vi "Meas 2 Target.vi"(7 "Cartesian Type":bool caption="CartesianType", 9 "LBCB 2  Data":T1, 10 "LBCB 1  Data":T1, 11 "Target":T2) -> (3 "Measured Value":T2)   [LabVIEW 2009]
uses:
  Target.ctl
  Data Access Objects/Metadata/LBCB Number.ctl
  Mixed Mode Cartesian Data.ctl
  Global Data/Cartesian Measurment Actions.ctl
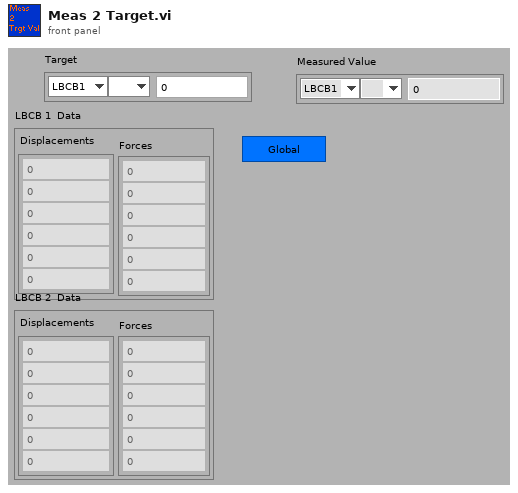
[diagram p1: front panel]
types:
  T1 = typedef "Mixed Mode Cartesian Data.ctl" = cluster{"Displacements":dbl[], "Forces":dbl[]}
  T2 = typedef "Target.ctl" = cluster{"LBCB Number":T3, "DOF Vectors":enum16{" ", "Dx", "Dy", "Dz", "Rx", "Ry", "Rz", "Fx", "Fy", "Fz", "Mx", "My", "Mz"}, "Amount":dbl}
  T3 = typedef "LBCB Number.ctl" = enum16{"LBCB1", "LBCB2"}
  T4 = typedef "Cartesian Measurment Actions.ctl" = enum16{"Set Data", "Get", "Init", "Set Offsets"}
  T5 = enum16{" ", "Dx", "Dy", "Dz", "Rx", "Ry", "Rz", "Fx", "Fy", "Fz", "Mx", "My", "Mz"}
  T6 = typedef "Cartesian Data Type.ctl" = cluster{"Displacements":dbl[], "Forces":dbl[], "Displacement Commands":dbl[]}
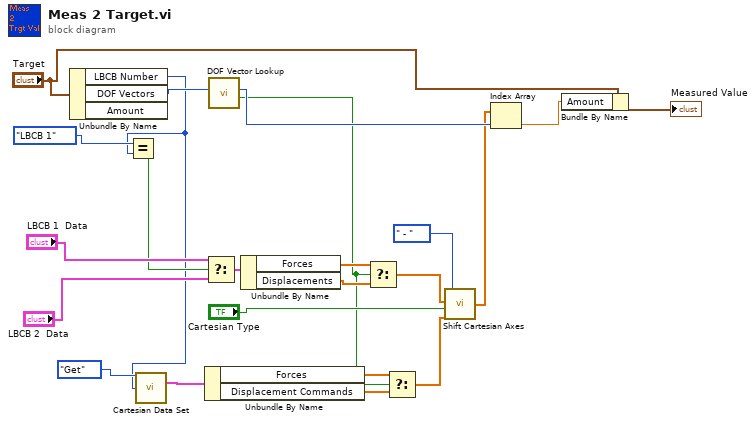
[diagram p0: block diagram]
diagram:
  n1 = Unbundle By Name("Target") -> ("LBCB Number"=w2:T3, "DOF Vectors"=w23:T5)  [unwired: 1 out]
  n2 = Equal?(x=enum16{"LBCB 1", "LBCB 2"}."LBCB 1", y=w2) -> (x = y?=w20:bool)
  n3 = call "Cartesian Data Set.vi"("Measurement Actions"=Cartesian_Measurment_Actions."Get", "LBCB Selected"=w2) -> ("Cartesian Data Offsets Out"=w1:T6)  [unwired: 4 in, 9 out]
  n4 = Unbundle By Name(w1) -> ("Forces"=w6:dbl[], "Displacement Commands"=w5:dbl[])
  n5 = Select(t="LBCB 1  Data", s=w20, f="LBCB 2  Data") -> (s? t:f=w16:T1)
  n6 = call "DOF Vector Lookup.vi"("DOF Vectors"=w23) -> ("IsForce"=w4:bool, "Index"=w17:u32)  [unwired: 9 out]
  n7 = Unbundle By Name(w16) -> ("Forces"=w15:dbl[], "Displacements"=w14:dbl[])
  n8 = Select(t=w15, s=w4, f=w14) -> (s? t:f=w12:dbl[])
  n9 = Select(t=w6, s=w4, f=w5) -> (s? t:f=w3:dbl[])
  n10 = call "Shift Cartesian Axes.vi"("Coordianate Offset"=w3, "Coordinate Switch"="Cartesian Type", "Coordianate Input"=w12, "Direction"=enum16{" +", " - "}." - ") -> ("Coordianate Output"=w11:dbl[])
  n11 = Index Array(array=w11, index=w17) -> (element=w13:dbl)
  n12 = Bundle By Name(cluster="Target", "Amount"=w13) -> (→"Measured Value":T2)
